vi "Static.Measure.Digital.vi"(10 "State":bool, 11 "Settings":T2={"ACTIVE EDGE"=TRUE}) -> (3 "Measurement":T1)   [LabVIEW 2015, in "Speciality FPGA IO.lvlib"]
uses:
  VeriStand FPGA Generation Wizard/Source/SubModules/FPGA Addon Speciality IO/Source/Speciality FPGA IO.lvlib
  Types/Static.Measure.Digital.Settings.ctl
  Types/Static.Measure.Digital.Measurement.ctl
  <vilib>/rvi/Emulation/niFpgaSctlEmulationGetInTimedLoop.vi
  <vilib>/rvi/Emulation/niFpgaProcessEmulError.vi
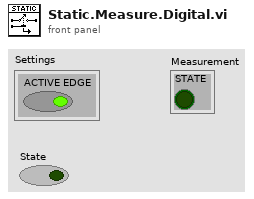
[diagram p1: front panel]
types:
  T1 = typedef "Speciality FPGA IO.lvlib/Static.Measure.Digital.Measurement.ctl" = cluster{"STATE":bool}
  T2 = typedef "Speciality FPGA IO.lvlib/Static.Measure.Digital.Settings.ctl" = cluster{"ACTIVE EDGE":bool}
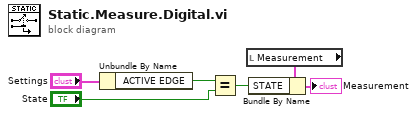
[diagram p0: block diagram]
diagram:
  n1 = Unbundle By Name("Settings") -> ("ACTIVE EDGE"=w5:bool)
  n2 = Equal?(x=w5, y="State") -> (x = y?=w3:bool)
  n3 = local read "Measurement"() -> (w1:T1)
  n4 = Bundle By Name(cluster=w1, "STATE"=w3) -> (→"Measurement":T1)
